vi "Converter_sample_is_in_selected_time.vi"(2 "enable VI input (T)":bool=TRUE, 5 "time format set":enum16{"LW_Data_Log-string", "SD-log-number"}(ring), 7 "Time in from csv":string, 10 "Time to":string, 11 "Time from":string) -> (3 "Is in time bounds?":bool)   [LabVIEW 2013]
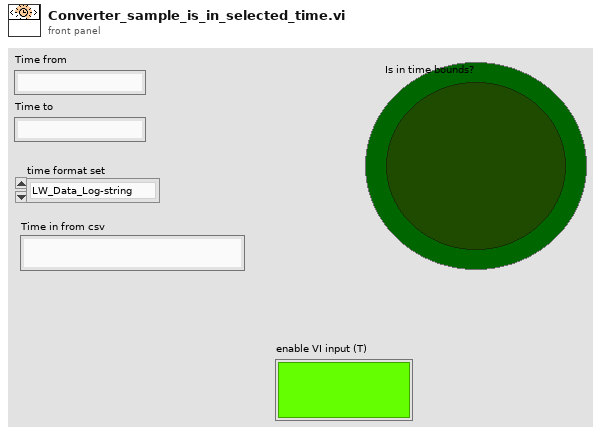
[diagram p1: front panel]
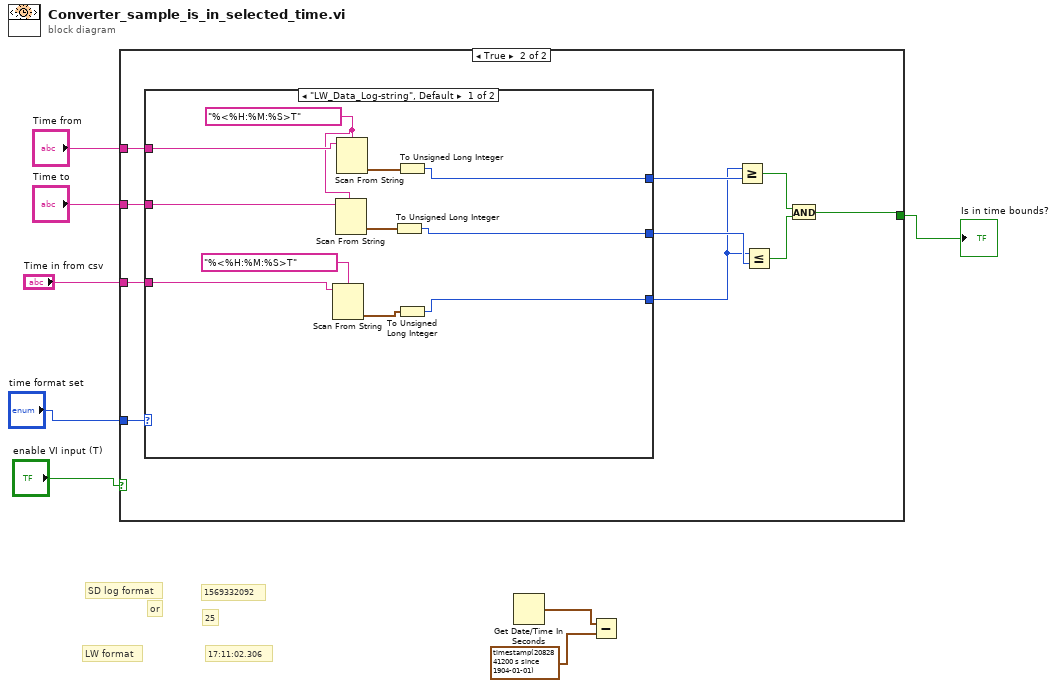
[diagram p0: block diagram]
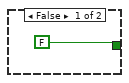
[diagram p2: hidden frame]
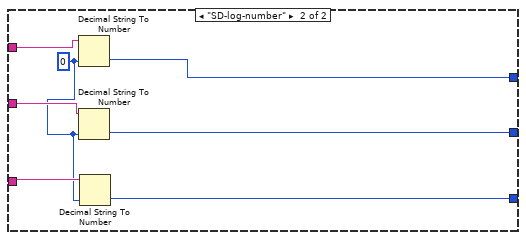
[diagram p3: hidden frame]
diagram:
  # "LW format"
  # "17:11:02.306"
  # "or"
  # "25"
  # "SD log format"
  # "1569332092"
  n1 = case shown="True" "enable VI input (T)" {
    tunnel: "time format set" -> [_ w19]
    tunnel: "Time in from csv" -> [_ w18]
    tunnel: "Time from" -> [_ w17]
    tunnel: "Time to" -> [_ w16]
    tunnel: [FALSE w10] -> w4
    frame False {
    }
    frame True {
      n2 = case shown="\"LW_Data_Log-string\", Default" w19 {
        tunnel: w18 -> [w29 w35]
        tunnel: w17 -> [w28 w37]
        tunnel: w16 -> [w27 w36]
        tunnel: [w22 w33] -> w13
        tunnel: [w21 w32] -> w12
        tunnel: [w20 w31] -> w11
        frame "LW_Data_Log-string", Default {
          w26 = "%<%H:%M:%S>T"
          n3 = Scan From String(format string="%<%H:%M:%S>T", input string=w29) -> (output 1=w25:timestamp)  [unwired: 3 in, 3 out]
          n4 = Scan From String(format string=w26, input string=w27) -> (output 1=w24:timestamp)  [unwired: 3 in, 3 out]
          n5 = Scan From String(format string=w26, input string=w28) -> (output 1=w23:timestamp)  [unwired: 3 in, 3 out]
          n6 = To Unsigned Long Integer(number=w24) -> (unsigned 32bit integer=w21:u32)
          n7 = To Unsigned Long Integer(number=w23) -> (unsigned 32bit integer=w22:u32)
          n8 = To Unsigned Long Integer(number=w25) -> (unsigned 32bit integer=w20:u32)
        }
        frame "SD-log-number" {
          w34 = u32 0 ("default (0 I32)")
          n9 = Decimal String To Number(string=w37, default (0L)=w34) -> (number=w33:u32)  [unwired: 1 in, 1 out]
          n10 = Decimal String To Number(string=w36, default (0L)=w34) -> (number=w32:u32)  [unwired: 1 in, 1 out]
          n11 = Decimal String To Number(string=w35, default (0L)=w34) -> (number=w31:u32)  [unwired: 1 in, 1 out]
        }
      }
      n12 = Greater Or Equal?(x=w11, y=w13) -> (x >= y?=w14:bool)
      n13 = Less Or Equal?(x=w11, y=w12) -> (x <= y?=w15:bool)
      n14 = And(x=w14, y=w15) -> (x .and. y?=w10:bool)
    }
  }
  "Is in time bounds?" <- w4
  n15 = Get Date/Time In Seconds() -> (seconds since 1Jan1904=w3:timestamp)
  n16 = Subtract(x=w3, y=timestamp(2082841200 s since 1904-01-01) ("current time")) -> ()  [unwired: 1 out]
